vi "CCC Client Init.vi"(8 "error in (no error)":errorcluster, 9 "Port (54444)":u16=54444, 10 "Server IP Address":string, 11 "CCC Tag List":T4[](array[typedef])) -> (0 "error out":errorcluster, 3 "CCC Connection ID":T1)   [LabVIEW 2010]
doc: "This VI is used by the client side of the CVT Client Communication API to initiate a connection with the server."
uses:
  ccc_TagConfiguration.ctl
  <vilib>/NI/Current Value Table/Compatibility/_SubVIs/TypeDefs/cvt_Data Types.ctl
  ccc_TagDirection.ctl
  ccc_ConnectionID.ctl
  <vilib>/NI/STM/compatibility/stm_TCP Connection Info.ctl
  <vilib>/NI/STM/compatibility/stm_MetaDataElement.ctl
  ccc_Convert To Compatibility TagConfig.vi
  NI_CCC.lvlib
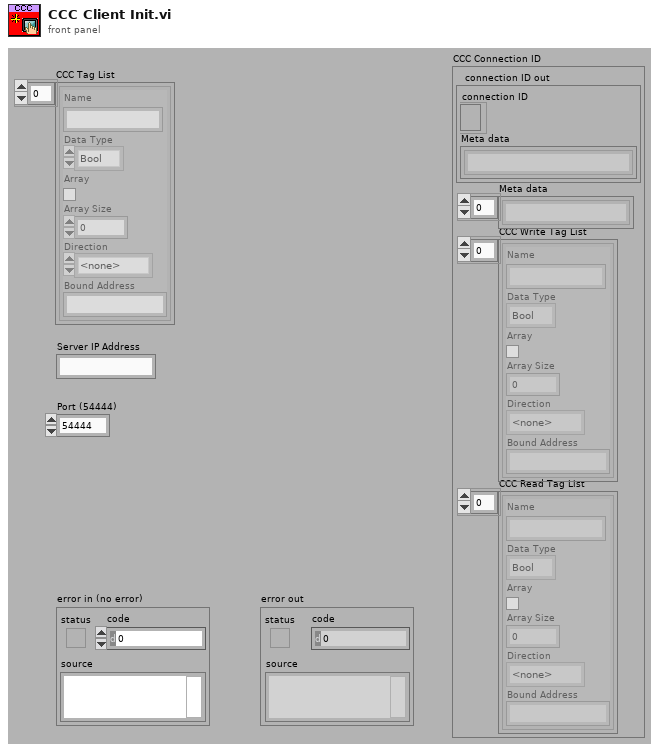
[diagram p1: front panel]
types:
  T1 = typedef "ccc_ConnectionID.ctl" = cluster{"connection ID out":T2, "Meta data":T3[], "CCC Write Tag List":T4[], "CCC Read Tag List":T4[]}
  T2 = typedef "stm_TCP Connection Info.ctl" = cluster{"connection ID":refnum<k5>, "Meta data":T3[]}
  T3 = typedef "stm_MetaDataElement.ctl" = string
  T4 = typedef "ccc_TagConfiguration.ctl" = cluster{"Name":string, "Data Type":T5, "Array":bool, "Array Size":u32, "Direction":T6, "Bound Address":string}
  T5 = typedef "cvt_Data Types.ctl" = enum16{"Bool", "U8", "I32", "Double", "String", "Enum"}
  T6 = typedef "ccc_TagDirection.ctl" = enum32{"<none>", "Read", "Write"}
  T7 = typedef "NI_CCC.lvlib/Tag Configuration.ctl" = cluster{"name":string, "data type":T8, "direction":T9, "bound address":string}
  T8 = typedef "Current Value Table.lvlib/Data Types.ctl" = enum16{"Double", "Single", "I64", "I32", "I16", "I8", "U64", "U32", "U16", "U8", "String", "Boolean", "Array of U8", "Array of U16", "Array of U32", "Array of U64", "Array of I64", "Array of I32", "Array of I16", "Array of I8", "Array of Double", "Array of Single", "Array of Boolean", "Array of String"}
  T9 = typedef "NI_CCC.lvlib/Tag Direction.ctl" = enum32{"<none>", "Read", "Write"}
  T10 = typedef "NI_CCC.lvlib/Connection ID.ctl" = cluster{"server ID":string, "connection ID":T11, "meta data":T12[], "write tag list":T7[], "read tag list":T7[]}
  T11 = typedef "NI STM.lvlib/TCP Connection Info.ctl" = cluster{"connection ID":refnum<k5>, "meta data":T12[]}
  T12 = typedef "NI STM.lvlib/MetaDataElement.ctl" = string
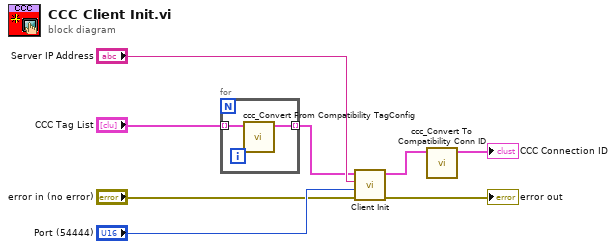
[diagram p0: block diagram]
diagram:
  n1 = for {
    tunnel: "CCC Tag List" -> [w10] mode=indexing
    tunnel: [w9] -> w1 mode=indexing
    n2 = call "ccc_Convert From Compatibility TagConfig.vi"("old tag"=w10) -> ("new tag"=w9:T7)  [unwired: 10 in]
  }
  n3 = call "Client Init.vi"("error in"="error in (no error)", "remote port (54444)"="Port (54444)", "server IP address"="Server IP Address", "tag list"=w1) -> ("error out"=→"error out":errorcluster, "connection ID"=w4:T10)  [unwired: 6 in]
  n4 = call "ccc_Convert To Compatibility Conn ID.vi"("new connection ID"=w4) -> ("old connection ID"=→"CCC Connection ID":T1)  [unwired: 10 in]
